vi "Track Goal.vi"(6 "Offset":dbl, 7 "Original Image":T3(plugin-control), 9 "Camera Type":T4, 10 "Targets":T5(array[cluster]), 11 "Goal Display":T3(plugin-control)) -> (0 "Angle Difference":dbl, 1 "Target Line Masking Out":T3(plugin-control), 2 "Best Target Available":T2, 3 "Found Targets":T6(array[cluster]) {"Normalized Rect"."Numeric 5" format="%#_2g"; "Normalized Rect"."Numeric 3" format="%#_2g"; "Normalized Rect"."Numeric 2" format="%#_2g"; "Normalized Rect"."Numeric" format="%#_2g"}, 5 "Goal Display":T3(plugin-control))   [LabVIEW 2015]
uses:
  Camera Types.ctl
panel:
  out "Sorted Scores":T1(array[cluster]) {"Moment Factor" format="%#_3g"; "L" format="%#_3g"; "Area to CH" format="%#_3g"; "X" format="%#_3g"; "Y" format="%#_3g"}
  # "Aspect Ratio"
  # "Density Profile"
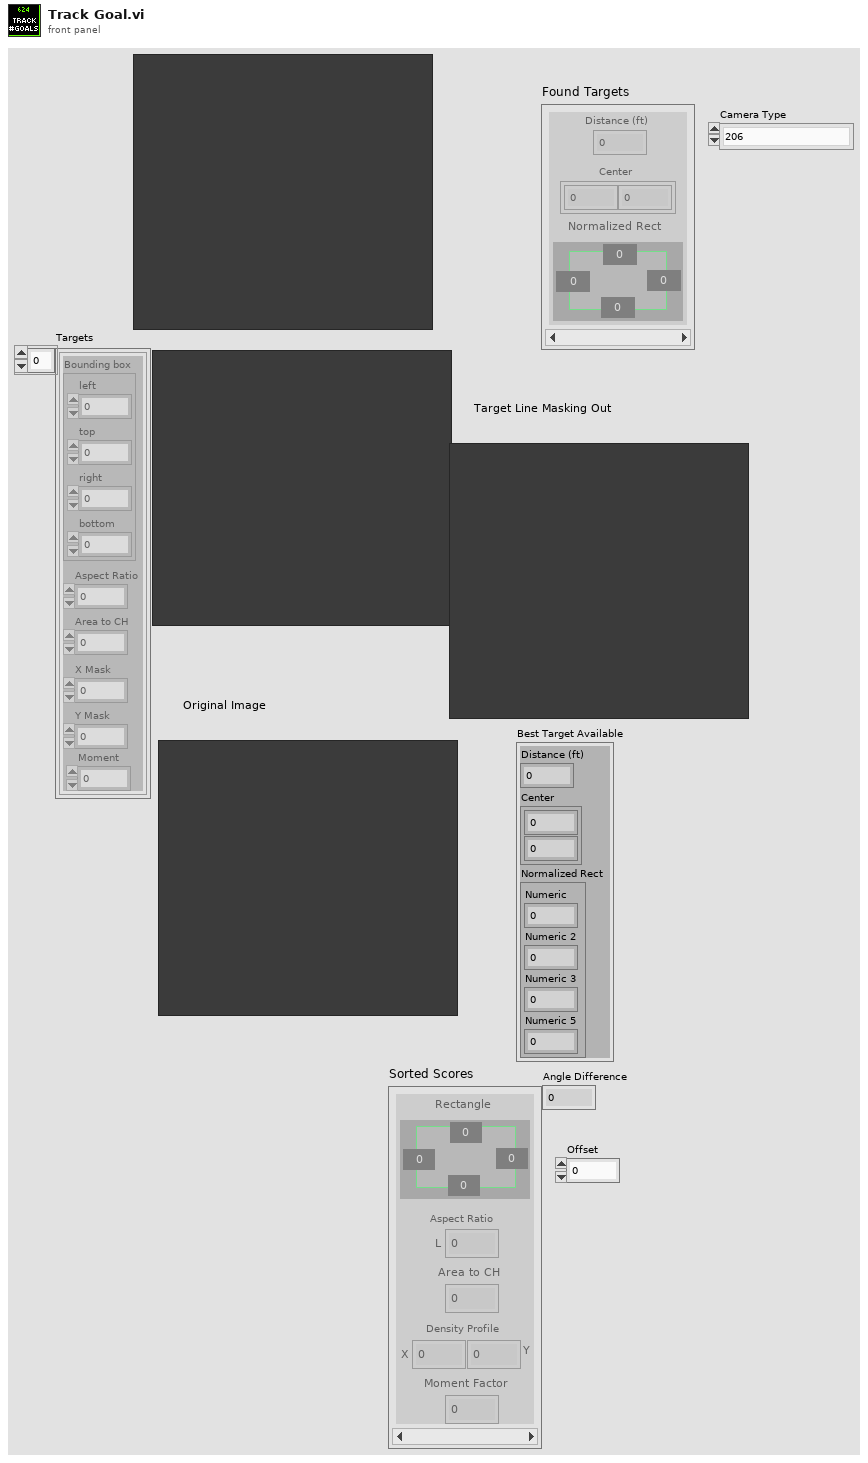
[diagram p1: front panel]
types:
  T1 = cluster{"Rectangle":cluster{"Numeric":dbl, "Numeric 2":dbl, "Numeric 3":dbl, "Numeric 5":dbl}, "L":dbl, "Area to CH":dbl, "X":dbl, "Y":dbl, "Moment Factor":dbl}[]
  T2 = cluster{"Distance (ft)":dbl, "Center":cluster{dbl, dbl}, "Normalized Rect":cluster{"Numeric":dbl, "Numeric 2":dbl, "Numeric 3":dbl, "Numeric 5":dbl}}
  T3 = typedef "IMAQ Image.ctl" = refnum<image>
  T4 = typedef "Camera Types.ctl" = enum16{"206", "1011", "1013", "MS HD3000 square", "MS HD3000 640x480"}
  T5 = cluster{"Bounding box":cluster{"left":dbl, "top":dbl, "right":dbl, "bottom":dbl}, "Aspect Ratio":dbl, "Area to CH":dbl, "X Mask":dbl, "Y Mask":dbl, "Moment":dbl}[]
  T6 = cluster{"Distance (ft)":dbl, "Center":cluster{dbl, dbl}, "Normalized Rect":cluster{"Numeric":dbl, "Numeric 2":dbl, "Numeric 3":dbl, "Numeric 5":dbl}}[]
  T7 = cluster{"Numeric":dbl, "Numeric 2":dbl, "Numeric 3":dbl, "Numeric 5":dbl}
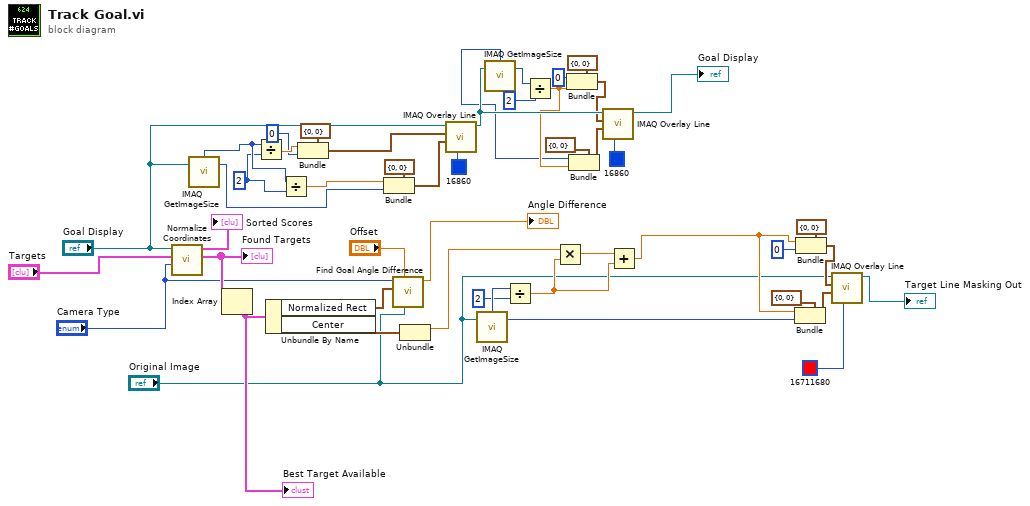
[diagram p0: block diagram]
diagram:
  w38 = 2 ("y")
  n1 = call "Normalize Coordinates.vi"("Camera Type"="Camera Type", "Targets"="Targets", "Image in"="Goal Display") -> ("Found Targets"=w16:T6, "Sorted Scores"=→"Sorted Scores":T1)  [unwired: 7 in]
  "Found Targets" <- w16
  n2 = call "IMAQ GetImageSize"("Image"="Goal Display") -> ("Y Resolution"=w36:i32, "X Resolution"=w39:i32)  [unwired: 3 in, 1 out]
  n3 = Index Array(array=w16) -> (element=w15:T2)  [unwired: 1 in]
  "Best Target Available" <- w15
  n4 = Divide(x=w39, y=w38) -> (x/y=w44:dbl)
  n5 = Unbundle By Name(w15) -> ("Normalized Rect"=w5:T7, "Center"=w14:cluster{dbl, dbl})
  n6 = Divide(x=w39, y=w38) -> (x/y=w42:dbl)
  n7 = Bundle(cluster=cluster{"X":i32, "Y":i32} {"X"=0, "Y"=0} ("Start Point"), "X"=w44, "Y"=0) -> (w40:cluster{"X":i32, "Y":i32})
  n8 = Bundle(cluster=cluster{"X":i32, "Y":i32} {"X"=0, "Y"=0} ("Start Point"), "X"=w42, "Y"=w36) -> (w37:cluster{"X":i32, "Y":i32})
  n9 = call "Find Goal Angle Difference.vi"("Goal Display 2"="Original Image", "Offset"="Offset", "Normalized Rect"=w5, "Camera Type"="Camera Type") -> ("Angle Diff"=→"Angle Difference":dbl)  [unwired: 7 in]
  n10 = Unbundle(w14) -> (w10:dbl)  [unwired: 1 out]
  n11 = call "IMAQ Overlay Line"("Color"=u32 16860, "End Point"=w37, "Start Point"=w40, "Image"="Goal Display") -> ("Image Out"=w35:T3)  [unwired: 6 in, 1 out]
  n12 = call "IMAQ GetImageSize"("Image"="Original Image") -> ("Y Resolution"=w17:i32, "X Resolution"=w12:i32)  [unwired: 3 in, 1 out]
  n13 = call "IMAQ GetImageSize"("Image"=w35) -> ("Y Resolution"=w33:i32, "X Resolution"=w26:i32)  [unwired: 3 in, 1 out]
  n14 = Divide(x=w12, y=2) -> (x/y=w8:dbl)
  n15 = Divide(x=w33, y=2) -> (x/y=w27:dbl)
  n16 = Multiply(x=w10, y=w8) -> (x*y=w9:dbl)
  n17 = Bundle(cluster=cluster{"X":i32, "Y":i32} {"X"=0, "Y"=0} ("Start Point"), "X"=0, "Y"=w27) -> (w28:cluster{"X":i32, "Y":i32})
  n18 = Bundle(cluster=cluster{"X":i32, "Y":i32} {"X"=0, "Y"=0} ("Start Point"), "X"=w26, "Y"=w27) -> (w25:cluster{"X":i32, "Y":i32})
  n19 = call "IMAQ Overlay Line"("Color"=u32 16860, "End Point"=w25, "Start Point"=w28, "Image"=w35) -> ("Image Out"=→"Goal Display":T3)  [unwired: 6 in, 1 out]
  n20 = Add(x=w9, y=w8) -> (x+y=w7:dbl)
  n21 = Bundle(cluster=cluster{"X":i32, "Y":i32} {"X"=0, "Y"=0} ("Start Point"), "X"=w7, "Y"=w17) -> (w22:cluster{"X":i32, "Y":i32})
  n22 = Bundle(cluster=cluster{"X":i32, "Y":i32} {"X"=0, "Y"=0} ("Start Point"), "X"=w7, "Y"=0 ("X")) -> (w21:cluster{"X":i32, "Y":i32})
  n23 = call "IMAQ Overlay Line"("Color"=u32 16711680, "End Point"=w22, "Start Point"=w21, "Image"="Original Image") -> ("Image Out"=→"Target Line Masking Out":T3)  [unwired: 6 in, 1 out]
